vi "HMI_Cluster.vi"() -> (2 "HMI Data Cluster":T1)   [LabVIEW 2019]
uses:
  Sub-VIs/Globals and Definitions/HMI Typedef.ctl
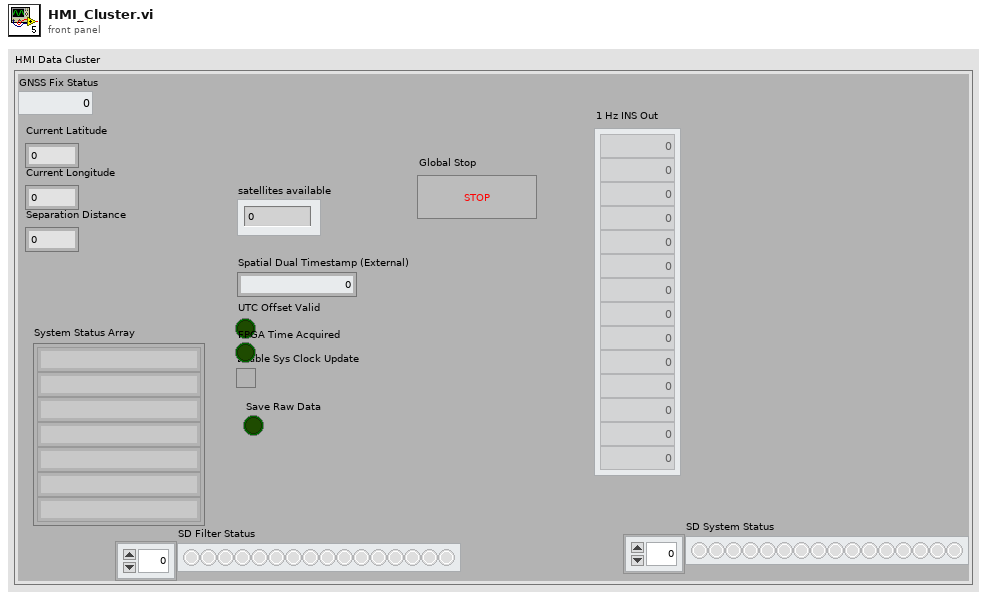
[diagram p1: front panel]
types:
  T1 = typedef "HMI Typedef.ctl" = cluster{"Current Latitude":dbl, "Current Longitude":dbl, "Separation Distance":dbl, "Global Stop":bool, "UTC Offset Valid":bool, "1 Hz INS Out":dbl[], "GNSS Fix Status":u32, "satellites available":u8, "System Status Array":string[], "Enable Sys Clock Update":bool, "Spatial Dual Timestamp (External)":u64, "SD Filter Status":bool[], "SD System Status":bool[], "FPGA Time Acquired":bool, "Save Raw Data":bool}
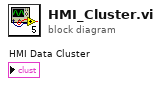
[diagram p0: block diagram]
diagram:
